vi "user initialization.vi"(8 "error in":errorcluster, 10 "configuration in":refnum<class "control module configuration.lvclass">, 11 "Watchdog runtime in":refnum<class "Watchdog runtime.lvclass">) -> (0 "error out":errorcluster, 3 "Watchdog runtime out":refnum<class "Watchdog runtime.lvclass">)   [LabVIEW 2013, in "Watchdog runtime.lvclass"]
uses:
  Watchdog runtime.lvclass
  <vilib>/NI/DCAF/Tag Editor Core/control module/configuration/control module configuration.lvclass
  configuration/Watchdog configuration.lvclass
  <vilib>/NI/DCAF/Tag Editor Core/control module/runtime/control module runtime.lvclass
  Watchdog runtime.lvclass/Watchdog runtime.ctl
  <vilib>/RTwatchdog.llb/Watchdog expiration actions.ctl
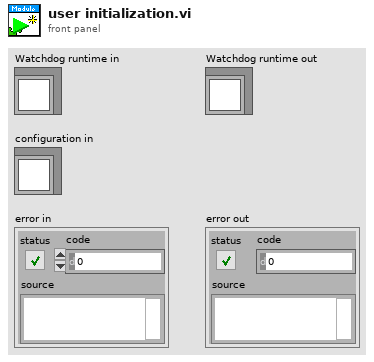
[diagram p1: front panel]
types:
  T1 = typedef "Watchdog expiration actions.ctl" = cluster{"reset":bool, "occurrence":bool, "trigger protocol":enum16{"active high", "active low", "open collector"}, "trigger line":enum16{"none", "line 0", "line 1", "line 2", "line 3", "line 4", "line 5", "line 6", "line 7", "SMB line 0"}, "disable watchdog on VI exit":bool}
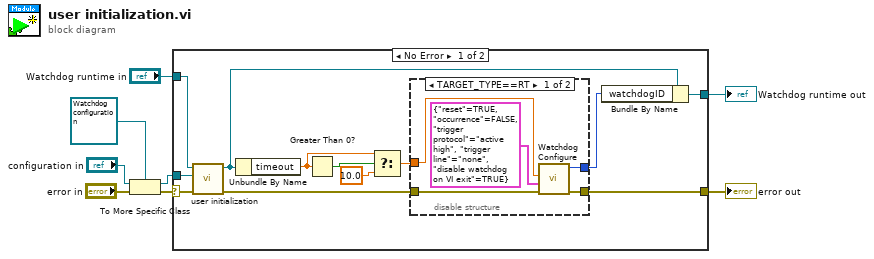
[diagram p0: block diagram]
diagram:
  n1 = To More Specific Class(target class=refnum<class "Watchdog configuration.lvclass"> refnum ("user module configuration"), reference="configuration in", error in="error in") -> (specific class reference=w1:refnum<class "Watchdog configuration.lvclass">, error out=w5:errorcluster)
  n2 = case shown="No Error" w5 {
    selector: w5 -> [w17 w27]
    tunnel: [w14 w28] -> w4
    tunnel: "Watchdog runtime in" -> [w11 w28]
    tunnel: [w16 w27] -> w2
    tunnel: w1 -> [w9 _]
    frame No Error {
      n3 = call-parent "user initialization.vi"("error in"=w17, "configuration in"=w9, "fixed channel runtime in"=w11) -> ("error out"=w12:errorcluster, "fixed channel runtime out"=w10:refnum<class "Watchdog runtime.lvclass">)  [unwired: 7 in]
      n4 = Unbundle By Name(w10) -> ("timeout"=w19:dbl)
      n5 = Greater Than 0?(x=w19) -> (x > 0?=w20:bool)
      n6 = Select(t=w19, s=w20, f=10.0) -> (s? t:f=w15:dbl)
      n7 = disable-structure shown="TARGET_TYPE==RT" {
        disable-tunnel: w12 -> [w25 w26]
        disable-tunnel: [w24 w26] -> w16
        disable-tunnel: w15 -> [w23 _]
        disable-tunnel: [w22 _] -> w13
        frame condition #0 (active) {
          n8 = call <vilib>:"Watchdog Configure.vi"("error in (no error)"=w25, "expiration actions"=T1 {"reset"=TRUE, "occurrence"=FALSE, "trigger protocol"=enum."active high", "trigger line"=enum."none", "disable watchdog on VI exit"=TRUE}, "timeout (1 sec)"=w23) -> ("error out"=w24:errorcluster, "watchdogID"=w22:u32)  [unwired: 1 in, 2 out]
        }
        frame condition #1 {
        }
      }
      n9 = Bundle By Name(cluster=w10, "watchdogID"=w13) -> (w14:refnum<class "Watchdog runtime.lvclass">)
    }
    frame Error {
    }
  }
  "error out" <- w2
  "Watchdog runtime out" <- w4
